vi "Poll State From File.vi"(11 "match_id":string) -> (3 "state":string)   [LabVIEW 2025]
panel:
  out "error out":errorcluster
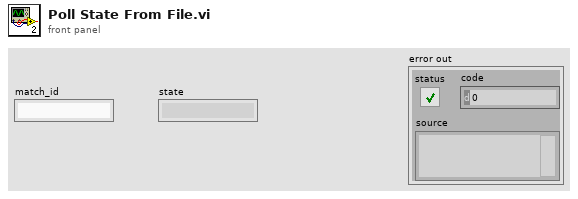
[diagram p1: front panel]
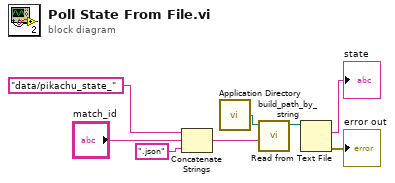
[diagram p0: block diagram]
diagram:
  n1 = Concatenate Strings("data/pikachu_state_" ("string"), "match_id", ".json" ("string")) -> (w5:string)
  n2 = call <vilib>:"Application Directory.vi"() -> ("Application Directory"=w6:path)
  n3 = call "build_path_by_string.vi"("String"=w5, "base path"=w6) -> ("appended path"=w8:path)  [unwired: 9 in]
  n4 = Read from Text File(file (use dialog)=w8) -> (text=→"state":string, error out=→"error out":errorcluster)  [unwired: 3 in, 2 out]
